vi "camara.vi"() -> ()   [LabVIEW 2020]
uses:
  <vilib>/userDefined/High Color/IMAQdx.ctl
  <vilib>/vision/driver/IMAQdx.llb/IMAQdx Buffer Number Mode.ctl
  <vilib>/vision/driver/NI_Vision_Acquisition_Software.lvlib
panel:
  in  "Buffer Number Mode (Next)":T1
  out "Image 2":T2(plugin-control)
  out "Image":T2(plugin-control)
  in  "Session In":T3
  in  "stop":bool
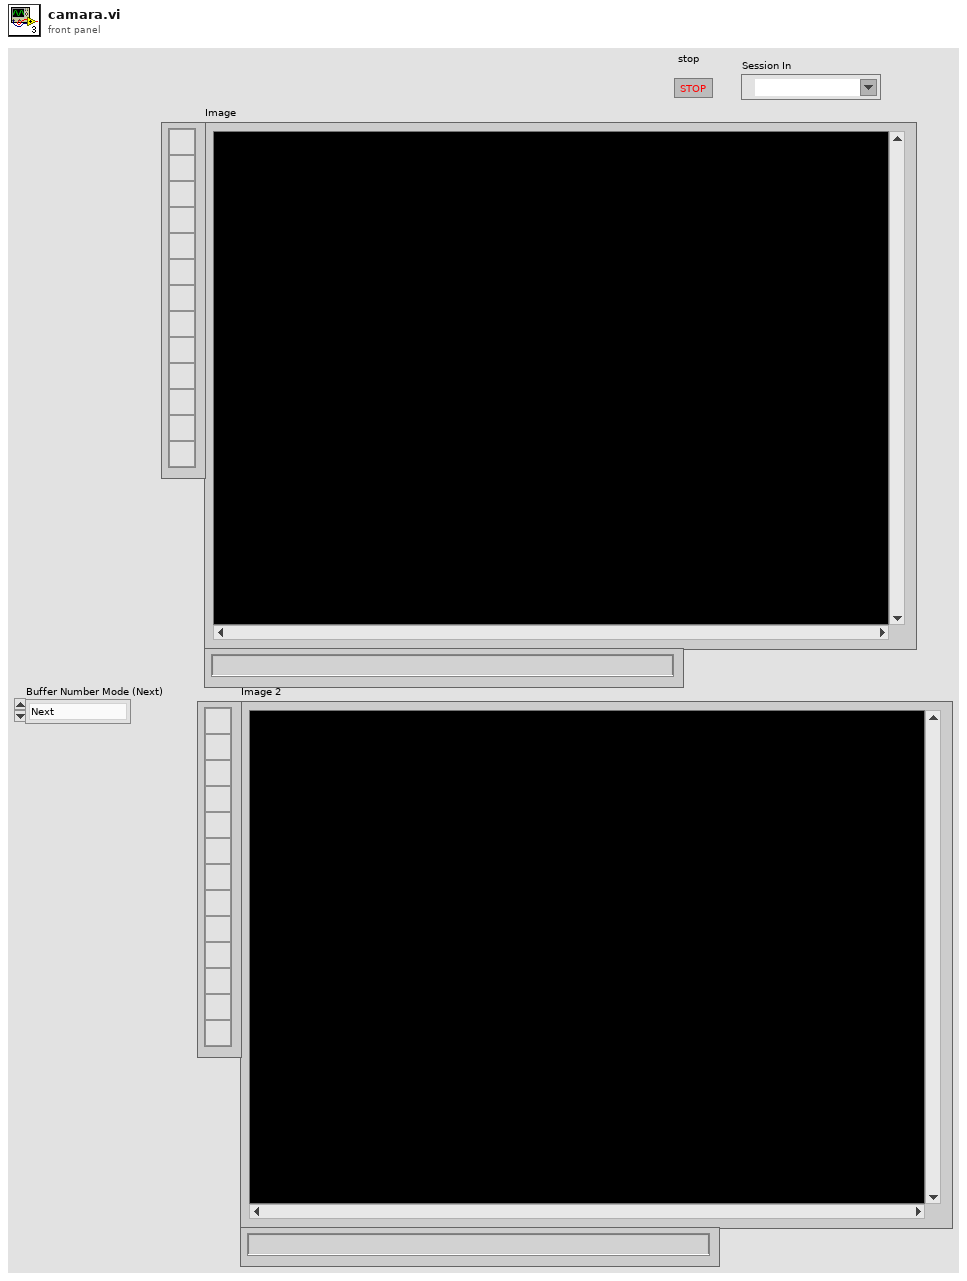
[diagram p1: front panel]
types:
  T1 = typedef "NI_Vision_Acquisition_Software.lvlib/IMAQdx Buffer Number Mode.ctl" = enum32{"Next", "Last", "Buffer Number", "Every", "Last New"}
  T2 = typedef "IMAQ Image.ctl" = refnum<image>
  T3 = typedef "IMAQdx.ctl" = refnum<k21>
  T4 = typedef "Image Type" = u32
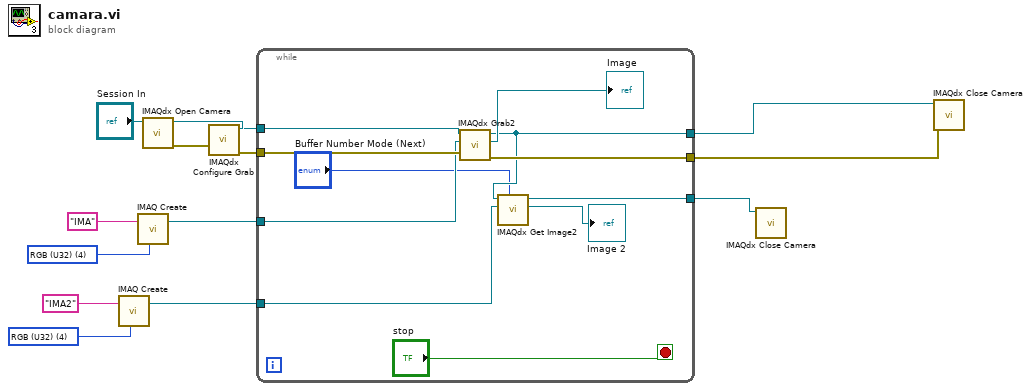
[diagram p0: block diagram]
diagram:
  w4 = T4 4 items=["Grayscale (U8)", "Grayscale (I16)", "Grayscale (SGL)", "Complex (CSG)", "RGB (U32)", "HSL (U32)", "RGB (U64)", "Grayscale (U16)"] ("Image Type")
  w6 = T4 4 items=["Grayscale (U8)", "Grayscale (I16)", "Grayscale (SGL)", "Complex (CSG)", "RGB (U32)", "HSL (U32)", "RGB (U64)", "Grayscale (U16)"] ("Image Type")
  n1 = call "IMAQ Create"("Image Name"="IMA2", "Image Type"=w4) -> ("New Image"=w2:T2)  [unwired: 3 in, 1 out]
  n2 = call "IMAQ Create"("Image Name"="IMA", "Image Type"=w6) -> ("New Image"=w5:T2)  [unwired: 3 in, 1 out]
  n3 = call <vilib>:"IMAQdx Open Camera.vi"("Session In"="Session In") -> ("error out"=w11:errorcluster, "Session Out"=w14:T3)  [unwired: 9 in]
  n4 = call <vilib>:"IMAQdx Configure Grab.vi"("error in"=w11, "Session In"=w14) -> ("error out"=w10:errorcluster, "Session Out"=w13:T3)  [unwired: 8 in]
  n5 = while {
    tunnel: w13 -> [w18]
    tunnel: [w16] -> w12
    tunnel: w10 -> [w24]
    tunnel: [w23] -> w9
    tunnel: w5 -> [w22]
    tunnel: w2 -> [w20]
    tunnel: [w17] -> w1
    stop <- "stop" stop-if-true
    n6 = call <vilib>:"IMAQdx Grab2.vi"("error in"=w24, "Image In"=w22, "Session In"=w18) -> ("error out"=w23:errorcluster, "Image Out"=→"Image":T2, "Session Out"=w16:T3)  [unwired: 5 in, 1 out]
    n7 = call <vilib>:"IMAQdx Get Image2.vi"("Buffer Number Mode (Next)"="Buffer Number Mode (Next)", "Image In"=w20, "Session In"=w16) -> ("Image Out"=→"Image 2":T2, "Session Out"=w17:T3)  [unwired: 5 in, 2 out]
  }
  n8 = call <vilib>:"IMAQdx Close Camera.vi"("Session In"=w1) -> ()  [unwired: 10 in, 1 out]
  n9 = call <vilib>:"IMAQdx Close Camera.vi"("error in"=w9, "Session In"=w12) -> ()  [unwired: 9 in, 1 out]
